vi "PostCopyScripting.vi"(10 "MetaDataObj":refnum<class "MetaDataObj.lvclass">, 11 "User Project":refnum<vi>) -> ()   [LabVIEW 2020, in "PluginMetaDataObj.lvclass"]
doc: "This VI renames all the necessary classes and libraries to the custom name."
uses:
  PluginMetaDataObj.lvclass
  <resource>/dialog/NewProjectWizard/MetaDataObj/MetaDataObj.lvclass
  C:/Program Files (x86)/National Instruments/LabVIEW 2020/resource/dialog/NewProjectWizard/MetaDataObj/MetaDataObj.lvclass
  <resource>/dialog/NewProjectWizard/MetaDataObj/MetaDataObj.lvclass/MetaDataObj.ctl
  <vilib>/Utility/EditLVProj/Edit LVProj.lvlib
  <resource>/dialog/NewProjectWizard/Project Copying/NI_NPW_Project Copying.lvlib
panel:
  out "error out":errorcluster
  in  "error in":errorcluster
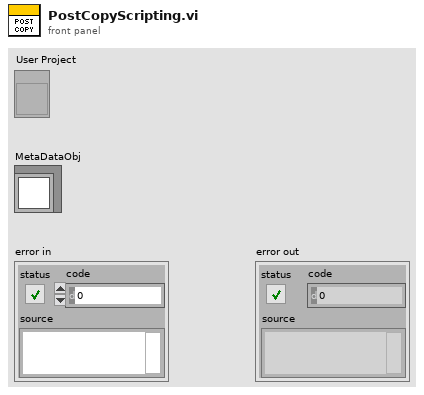
[diagram p1: front panel]
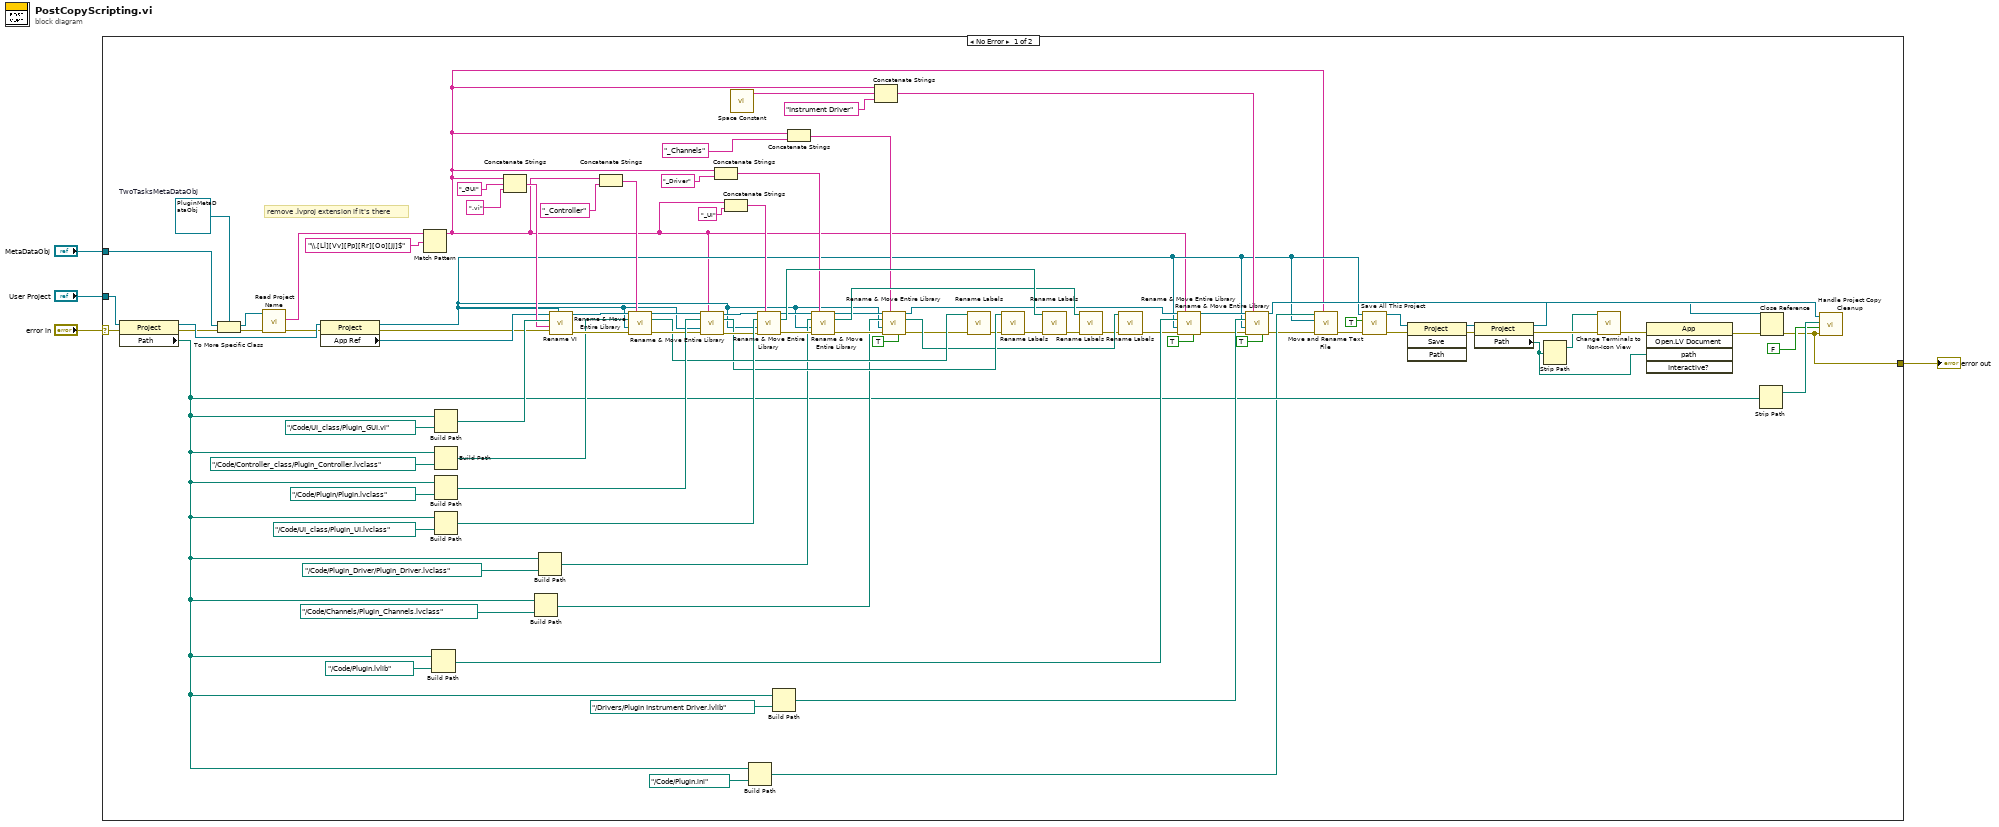
[diagram p0: block diagram]
diagram:
  n1 = case shown="No Error" "error in" {
    selector: "error in" -> [w29 w97]
    tunnel: "MetaDataObj" -> [w96 _]
    tunnel: "User Project" -> [w94 _]
    tunnel: [w30 w97] -> w1
    frame No Error {
      w95 = refnum<class "PluginMetaDataObj.lvclass"> refnum  # TwoTasksMetaDataObj
      # "remove .lvproj extension if it's there"
      n2 = property class="Project"(reference=w94, error in=w29) -> (reference out=w69:refnum<vi>, error out=w28:errorcluster, "Path"=w10:path)
      n3 = To More Specific Class(target class=w95, reference=w96, error in=w28) -> (specific class reference=w70:refnum<class "PluginMetaDataObj.lvclass">, error out=w68:errorcluster)
      n4 = call <resource>:"Read Project Name.vi"("error in (no error)"=w68, "MetaDataObj in"=w70) -> ("error out"=w67:errorcluster, "Project Name"=w71:string)  [unwired: 7 in, 1 out]
      n5 = property class="Project"(reference=w69, error in=w67) -> (reference out=w8:refnum<vi>, error out=w19:errorcluster, "App Ref"=w20:refnum<vi>)
      n6 = Match Pattern(string=w71, regular expression="\\.[Ll][Vv][Pp][Rr][Oo][Jj]$") -> (before substring=w5:string)  [unwired: 1 in, 3 out]
      n7 = Build Path(base path=w10, name or relative path=path "../Code/Plugin.lvlib" ("Path")) -> (appended path=w61:path)
      n8 = Build Path(base path=w10, name or relative path=path "../Code/UI_class/Plugin_GUI.vi" ("Path")) -> (appended path=w88:path)
      n9 = Build Path(base path=w10, name or relative path=path "../Code/Controller_class/Plugin_Controller.lvclass" ("Path")) -> (appended path=w60:path)
      n10 = Build Path(base path=w10, name or relative path=path "../Code/Plugin/Plugin.lvclass" ("Path")) -> (appended path=w72:path)
      n11 = Build Path(base path=w10, name or relative path=path "../Code/UI_class/Plugin_UI.lvclass" ("Path")) -> (appended path=w73:path)
      n12 = Concatenate Strings(w5, "_GUI" ("string"), ".vi" ("string")) -> (w75:string)
      n13 = Build Path(base path=w10, name or relative path=path "../Code/Channels/Plugin_Channels.lvclass" ("Path")) -> (appended path=w37:path)
      n14 = Build Path(base path=w10, name or relative path=path "../Code/Plugin_Driver/Plugin_Driver.lvclass" ("Path")) -> (appended path=w47:path)
      n15 = call "Rename VI.vi"("Project"=w8, "error in (no error)"=w19, "new vi name"=w75, "vi path"=w88, "Application"=w20) -> ("error out"=w87:errorcluster, "dup Application"=w86:refnum<vi>)  [unwired: 5 in]
      n16 = Concatenate Strings(w5, "_Controller" ("string")) -> (w64:string)
      n17 = call "Rename & Move Entire Library.vi"("Application"=w86, "New Name Without Extension"=w64, "Library Path"=w60, "Project"=w8, "error in"=w87) -> ("Application out"=w58:refnum<vi>, "New Library Path"=w55:path, "error out"=w59:errorcluster)  [unwired: 8 in]
      n18 = call "Rename & Move Entire Library.vi"("Application"=w58, "New Name Without Extension"=w5, "Library Path"=w72, "Project"=w8, "error in"=w59) -> ("Application out"=w56:refnum<vi>, "New Library Path"=w54:path, "error out"=w57:errorcluster)  [unwired: 8 in]
      n19 = Concatenate Strings(w5, "_Driver" ("string")) -> (w43:string)
      n20 = Concatenate Strings(w5, "_UI" ("string")) -> (w62:string)
      n21 = call <vilib>:"Space Constant.vi"() -> ("String"=w32:string)
      n22 = Build Path(base path=w10, name or relative path=path "../Code/Plugin.ini" ("Path")) -> (appended path=w9:path)
      n23 = call "Rename & Move Entire Library.vi"("Application"=w56, "New Name Without Extension"=w62, "Library Path"=w73, "Project"=w8, "error in"=w57) -> ("Application out"=w50:refnum<vi>, "New Library Path"=w53:path, "error out"=w49:errorcluster)  [unwired: 8 in]
      n24 = Build Path(base path=w10, name or relative path=path "../Drivers/Plugin Instrument Driver.lvlib" ("Path")) -> (appended path=w22:path)
      n25 = Concatenate Strings(w5, "_Channels" ("string")) -> (w40:string)
      n26 = call "Rename & Move Entire Library.vi"("Application"=w50, "New Name Without Extension"=w43, "Library Path"=w47, "Project"=w8, "error in"=w49) -> ("Application out"=w39:refnum<vi>, "New Library Path"=w46:path, "error out"=w42:errorcluster)  [unwired: 8 in]
      n27 = Concatenate Strings(w5, w32, "Instrument Driver" ("string")) -> (w25:string)
      n28 = call "Rename & Move Entire Library.vi"("Application"=w39, "New Name Without Extension"=w40, "Library Path"=w37, "Project"=w8, "error in"=w42, "Rename File only(T)"=TRUE ("Class(F) or Library(T)")) -> ("Application out"=w26:refnum<vi>, "New Library Path"=w36:path, "error out"=w27:errorcluster)  [unwired: 7 in]
      n29 = call "Rename Labels.vi"("error in"=w27, "Class Path"=w55) -> ("error out"=w52:errorcluster)  [unwired: 9 in]
      n30 = call "Rename Labels.vi"("error in"=w52, "Class Path"=w54) -> ("error out"=w51:errorcluster)  [unwired: 9 in]
      n31 = call "Rename Labels.vi"("error in"=w51, "Class Path"=w53) -> ("error out"=w45:errorcluster)  [unwired: 9 in]
      n32 = call "Rename Labels.vi"("error in"=w45, "Class Path"=w46) -> ("error out"=w35:errorcluster)  [unwired: 9 in]
      n33 = call "Rename Labels.vi"("error in"=w35, "Class Path"=w36) -> ("error out"=w34:errorcluster)  [unwired: 9 in]
      n34 = call "Rename & Move Entire Library.vi"("Application"=w26, "New Name Without Extension"=w5, "Library Path"=w61, "Project"=w8, "error in"=w34, "Rename File only(T)"=TRUE ("Class(F) or Library(T)")) -> ("Application out"=w24:refnum<vi>, "error out"=w21:errorcluster)  [unwired: 7 in, 1 out]
      n35 = call "Rename & Move Entire Library.vi"("Application"=w24, "New Name Without Extension"=w25, "Library Path"=w22, "Project"=w8, "error in"=w21, "Rename File only(T)"=TRUE ("Class(F) or Library(T)")) -> ("Application out"=w23:refnum<vi>, "error out"=w7:errorcluster)  [unwired: 7 in, 1 out]
      n36 = call "Move and Rename Text File.vi"("Project Name"=w5, "error in (no error)"=w7, "Project"=w8, "Template INI Path"=w9) -> ("error out"=w6:errorcluster)  [unwired: 7 in]
      n37 = call <vilib>:"Save All This Project.vi"("error in (no error)"=w6, "Exclude Dependencies? (F)"=TRUE, "Project in"=w8) -> ("error out"=w83:errorcluster, "Project out"=w81:refnum<vi>)  [unwired: 7 in]
      n38 = invoke class="Project" method="Save"(reference=w81, error in=w83) -> (reference out=w80:refnum<vi>, error out=w82:errorcluster)  [unwired: 2 in, 2 out]
      n39 = property class="Project"(reference=w80, error in=w82) -> (reference out=w79:refnum<vi>, error out=w18:errorcluster, "Path"=w16:path)
      n40 = Strip Path(path=w16) -> (stripped path=w15:path)  [unwired: 1 out]
      n41 = call "Change Terminals to Non-Icon View.vi"("error in"=w18, "Folder Path"=w15) -> ("error out"=w17:errorcluster)  [unwired: 9 in]
      n42 = invoke class="App" method="Open.LV Document"(error in=w17, "path"=w16) -> (error out=w85:errorcluster)  [unwired: 3 in, 4 out]
      n43 = Strip Path(path=w10) -> (stripped path=w78:path)  [unwired: 1 out]
      n44 = Close Reference(reference=w23, error in (no error)=w85) -> (error out=w30:errorcluster)
      n45 = call <resource>:"Handle Project Copy Cleanup.vi"("error in (no error)"=w30, "More Scripting?"=FALSE, "Target Path"=w78, "Project in"=w79) -> ()  [unwired: 8 in]
    }
    frame Error {
    }
  }
  "error out" <- w1
